vi "Read Dev Stream.vi"(8 "error in (no error)":errorcluster, 11 "VISA resource name":refnum<visa-resource-name>) -> (0 "error out":errorcluster, 2 "dev stream":u16(ring) items=["NORMAL", "ERROR"], 3 "VISA resource name out":refnum<visa-resource-name>)   [LabVIEW 2021, in "Andeen-Hagerling 2700A.lvlib"]
doc: "Return the state of the dev stream parameter.\n\nThe dev stream parameter is used to select whether the E (Error) or\nthe N (Normal) Data Stream will supply the results reported to\nthe front panel and remote devices as the result of executing\nthe SINGLE, CONTINUOUS, or FETCH commands while\nin the deviation mode."
uses:
  Andeen-Hagerling 2700A.lvlib
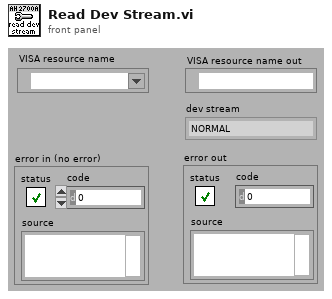
[diagram p1: front panel]
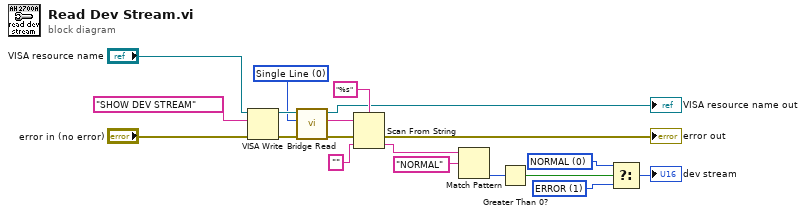
[diagram p0: block diagram]
diagram:
  w1 = u16 0 items=["Single Line", "Multi-Line"] ("Multiline")
  w8 = u16 0 items=["NORMAL", "ERROR"] ("dev stream (NORMAL)")
  w7 = u16 1 items=["NORMAL", "ERROR"] ("dev stream (NORMAL)")
  n1 = VISA Write(VISA resource name="VISA resource name", write buffer="SHOW DEV STREAM" ("command"), error in (no error)="error in (no error)") -> (VISA resource name out=w3:refnum<visa-resource-name>, error out=w2:errorcluster)  [unwired: 1 out]
  n2 = call "Bridge Read.vi"("error in (no error)"=w2, "multiline"=w1, "VISA resource name"=w3) -> ("error out"=w5:errorcluster, "read buffer"=w4:string, "VISA resource name out"=→"VISA resource name out":refnum<visa-resource-name>)  [unwired: 6 in]
  n3 = Scan From String(format string="%s", input string=w4, error in=w5, default 1="" ("default value 1")) -> (error out=→"error out":errorcluster, output 1=w12:string)  [unwired: 1 in, 2 out]
  n4 = Match Pattern(string=w12, regular expression="NORMAL") -> (offset past match=w11:i32)  [unwired: 1 in, 3 out]
  n5 = Greater Than 0?(x=w11) -> (x > 0?=w10:bool)
  n6 = Select(t=w8, s=w10, f=w7) -> (s? t:f=→"dev stream":u16)
